vi "RemoveEmptyRows2.vi"(8 "Error In":errorcluster, 11 "Array 3":string[](array[string])) -> (0 "Error Out":errorcluster, 3 "Array 4":string[](array[string]))   [LabVIEW 2014]
uses:
  <userlib>/_RADE/MTA-lib/array/array.llb/Search 1D Array (String)__ogtk.vi
  <userlib>/_RADE/MTA-lib/array/array.llb/Delete Elements from 1D Array (String)__ogtk.vi
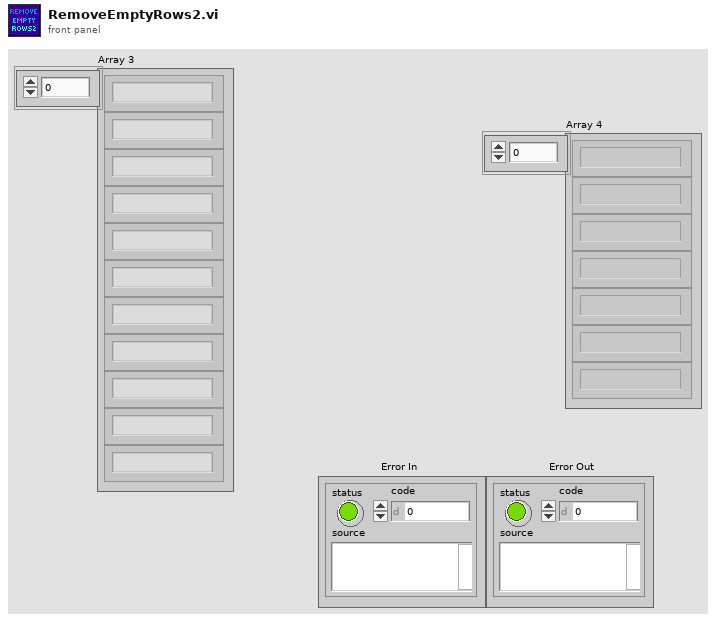
[diagram p1: front panel]
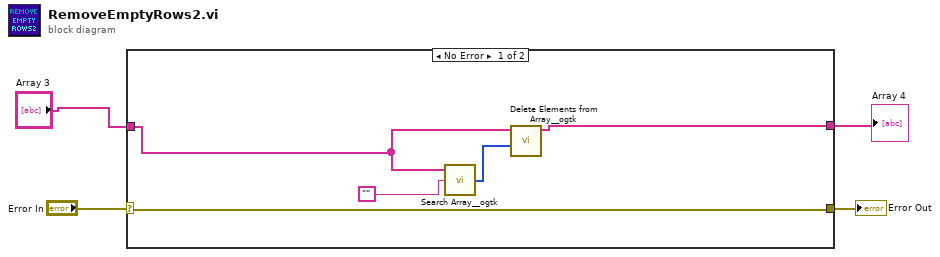
[diagram p0: block diagram]
diagram:
  n1 = case shown="No Error" "Error In" {
    selector: "Error In" -> [w9 w10]
    tunnel: [w5 w11] -> w1
    tunnel: "Array 3" -> [w6 w11]
    tunnel: [w9 w10] -> w3
    frame No Error {
      n2 = call-poly <userlib>:"Search Array__ogtk.vi"("Array"=w6, "Element Data"="") -> ("Indices of Elements"=w7:i32[])  [unwired: 7 in]
      n3 = call-poly <userlib>:"Delete Elements from Array__ogtk.vi"("indices"=w7, "array"=w6) -> ("array w/ subset deleted"=w5:string[])  [unwired: 8 in, 1 out]
    }
    frame Error {
    }
  }
  "Error Out" <- w3
  "Array 4" <- w1
